vi "initJuicer.vi"(8 "error in (no error)":errorcluster, 10 "Lines":string[](array[string])=["Dev3/port0/line0", "Dev3/port0/line1", "Dev3/port0/line2", "Dev3/port0/line3", "Dev3/port0/line4"], 11 "Juicer in":refnum<class "Juicer.lvclass">) -> (0 "error out":errorcluster, 3 "Juicer out":refnum<class "Juicer.lvclass">)   [LabVIEW 2014, in "Juicer.lvclass"]
uses:
  Juicer.lvclass
  Juicer.lvclass/Juicer.ctl
  <vilib>/DAQmx/create/channels.llb/DAQmx Create Channel (DO-Digital Output).vi
  <resource>/objmgr/daqmx.rc
panel:
  in  "Cluster":cluster{"Window Number (0...15)":i32}
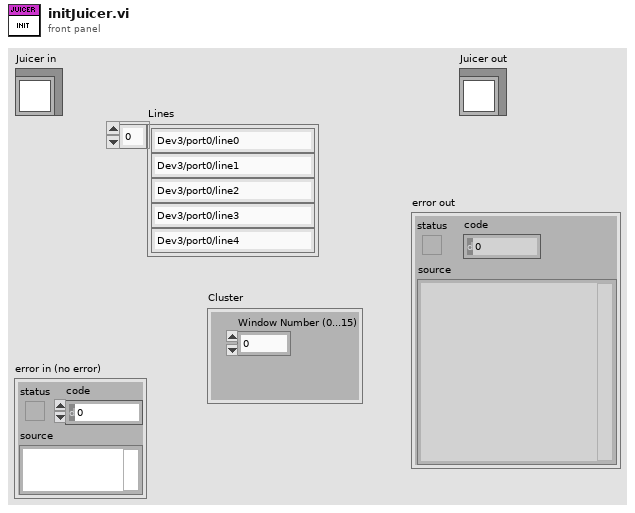
[diagram p1: front panel]
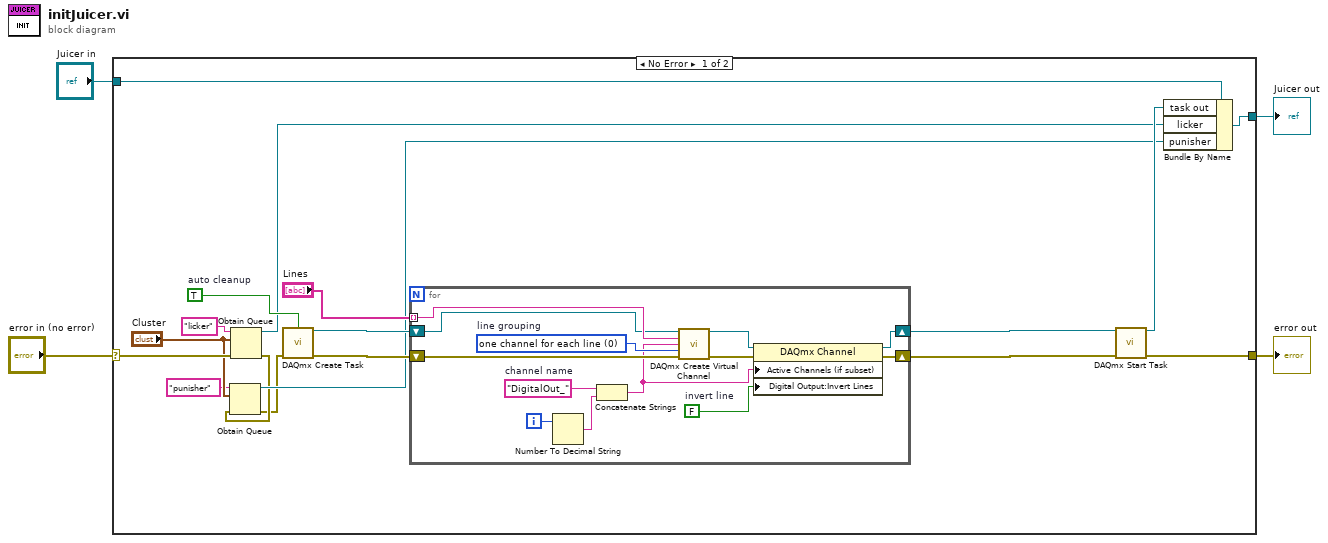
[diagram p0: block diagram]
diagram:
  n1 = case shown="No Error" "error in (no error)" {
    selector: "error in (no error)" -> [w13 w37]
    tunnel: [w18 w37] -> w3
    tunnel: [w21 w36] -> w1
    tunnel: "Juicer in" -> [w22 w36]
    frame No Error {
      w20 = TRUE  # auto cleanup
      n2 = Obtain Queue(name (unnamed)="licker", element data type="Cluster", error in (no error)=w13) -> (queue out=w12:refnum<queue>, error out=w6:errorcluster)  [unwired: 2 in, 1 out]
      n3 = Obtain Queue(name (unnamed)="punisher", element data type="Cluster", error in (no error)=w6) -> (queue out=w7:refnum<queue>, error out=w5:errorcluster)  [unwired: 2 in, 1 out]
      n4 = call <vilib>:"DAQmx Create Task.vi"("auto cleanup"=w20, "error in"=w5) -> ("task out"=w16:refnum<k21>, "error out"=w15:errorcluster)  [unwired: 12 in]
      n5 = for {
        tunnel: "Lines" -> [w31] mode=indexing
        shift-right: [w25] -> w11
        shift-left: w16 -> [w30]
        shift-right: [w24] -> w10
        shift-left: w15 -> [w28]
        i -> [w32]
        w29 = 0 items=["one channel for each line", "one channel for all lines"]  # line grouping
        w34 = "DigitalOut_"  # channel name
        w35 = FALSE  # invert line
        n6 = Number To Decimal String(number=w32) -> (decimal integer string=w33:string)  [unwired: 1 in]
        n7 = Concatenate Strings(w34, w33) -> (w23:string)
        n8 = call-poly <vilib>:"DAQmx Create Virtual Channel.vi"("task in"=w30, "lines"=w31, "name to assign"=w23, "line grouping"=w29, "error in"=w28) -> ("task out"=w26:refnum<k21>, "error out"=w27:errorcluster)  [unwired: 9 in]
        n9 = property class="DAQmx Channel"(reference=w26, error in=w27, "Active Channels (if subset)"=w23, "Digital Output:Invert Lines"=w35) -> (reference out=w25:refnum<k21>, error out=w24:errorcluster)
      }
      n10 = call <vilib>:"DAQmx Start Task.vi"("task/channels in"=w11, "error in"=w10) -> ("task out"=w19:refnum<k21>, "error out"=w18:errorcluster)  [unwired: 12 in]
      n11 = Bundle By Name(cluster=w22, "task out"=w19, "licker"=w12, "punisher"=w7) -> (w21:refnum<class "Juicer.lvclass">)
    }
    frame Error {
    }
  }
  "error out" <- w3
  "Juicer out" <- w1
